vi "PCI Configuration.Status.66 MHz Capable.Get.vi"(8 "error in (no error)":errorcluster, 11 "GE 5565PIORC":refnum<class "GE 5565PIORC.lvclass">) -> (0 "error out":errorcluster, 2 "66 MHz Capable?":bool, 3 "GE 5565PIORC out":refnum<class "GE 5565PIORC.lvclass">)   [LabVIEW 2016, in "GE 5565PIORC.lvclass"]
uses:
  GE 5565PIORC.lvclass
  GE 5565PIORC.lvclass/GE 5565PIORC.ctl
  <vilib>/Instr/_visa.llb/VISA Register Access Address Space.ctl
  Controls/Registers.PCI Configuration.ctl
  Binary Operations/Get Bits U16.vi
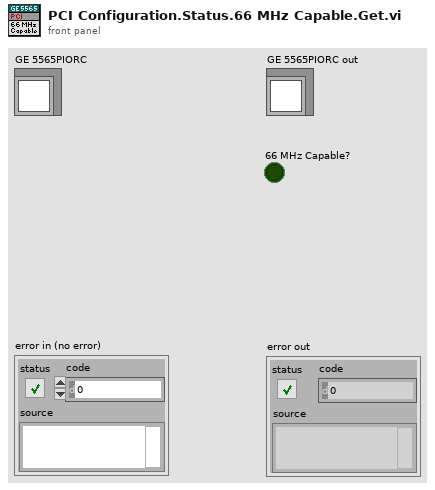
[diagram p1: front panel]
types:
  T1 = typedef "GE 5565PIORC.lvclass/Registers.PCI Configuration.ctl" = u32
  T2 = typedef "VISA Register Access Address Space.ctl" = u16
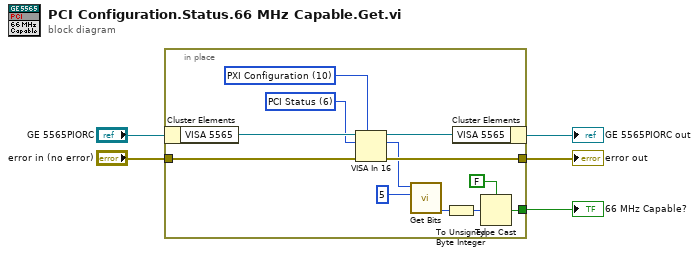
[diagram p0: block diagram]
diagram:
  n1 = in-place {
    in-place-border: "error in (no error)" -> [w15]
    in-place-border: [w14] -> w3
    in-place-border: [w6] -> w1
    w13 = T1 6 items=["PCI Configuration ID"=0, "PCI Command"=4, "PCI Status"=6, "PCI Revision ID"=8, "PCI Class Code"=9, "PCI Cache Line Size"=12, "PCI Latency Timer"=13, "PCI Header Type"=14, "PCI Built-In Self-Test"=15, "PCI BAR 0"=16, "PCI BAR 1"=20, "PCI BAR 2"=24, "PCI BAR 3"=28, "PCI BAR 4"=32, "PCI BAR 5"=36, "PCI Cardbus CIS Pointer"=40, "PCI Subsystem Vendor ID"=44, "PCI Subsytem ID"=46, "PCI Expansion ROM Base"=48, "PCI Capability Pointer"=52, "PCI Interrupt Line"=60, "PCI Interrupt Pin"=61, "PCI Min_Gnt"=62, "PCI Max_Lat"=63] ("PCI Configuration Register")
    w12 = T2 10 items=["VXI/VME A16"=1, "VXI/VME A24"=2, "VXI/VME A32"=3, "VXI/VME A64"=4, "PXI Memory Allocations"=9, "PXI Configuration"=10, "PXI BAR0"=11, "PXI BAR1"=12, "PXI BAR2"=13, "PXI BAR3"=14, "PXI BAR4"=15, "PXI BAR5"=16] ("Address Space")
    n2 = in-place-cluster #1("GE 5565PIORC") -> ("VISA 5565"=w17:refnum<visa-resource-name>)
    n3 = VISA In 16(7:w12, 8:w15, 10:w13, 11:w17) -> (0:w14:errorcluster, 2:w11:u16, 3:w16:refnum<visa-resource-name>)
    n4 = call-poly "Get Bits.vi"("Start Index (0)"=u8 5, "Register in"=w11) -> ("Value"=w7:u16)  [unwired: 6 in, 3 out]
    n5 = To Unsigned Byte Integer(number=w7) -> (unsigned 8bit integer=w8:u8)
    n6 = in-place-cluster #1("VISA 5565"=w16) -> (→"GE 5565PIORC out":refnum<class "GE 5565PIORC.lvclass">)
    n7 = Type Cast(type=FALSE, x=w8) -> (*(type *) &x=w6:bool)
  }
  "error out" <- w3
  "66 MHz Capable?" <- w1
